vi "copy Data to Array 2D.vi"(4 "error in (no error)":errorcluster, 7 "Data in":refnum<class "Data.lvclass">) -> (0 "error out":errorcluster, 2 "Data Content":sgl[][](array[numeric]), 3 "Data out":refnum<class "Data.lvclass">)   [LabVIEW 2017]
uses:
  C:/Program Files/Thorlabs/SpectralRadar/LabVIEW/2012/user.lib/SpectralRadar.llb/Data.lvclass
  C:/Program Files/Thorlabs/SpectralRadar/LabVIEW/2012/user.lib/SpectralRadar.llb/Data Property Int Selection.ctl
  C:/Program Files/Thorlabs/SpectralRadar/LabVIEW/2012/user.lib/SpectralRadar.llb/get Data Property Int.vi
  SpectralRadar.dll
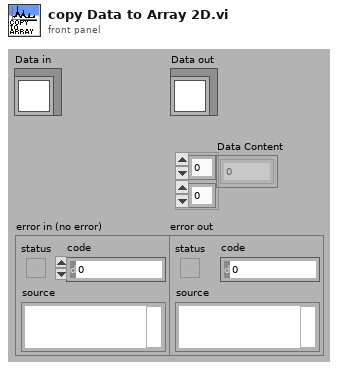
[diagram p1: front panel]
types:
  T1 = typedef "Data.lvclass/Data Property Int Selection.ctl" = enum16{"Dimensions", "Size 1", "Size 2", "Size 3", "Number of Data Points", "Data Size in Bytes", "Bytes per Pixel"}
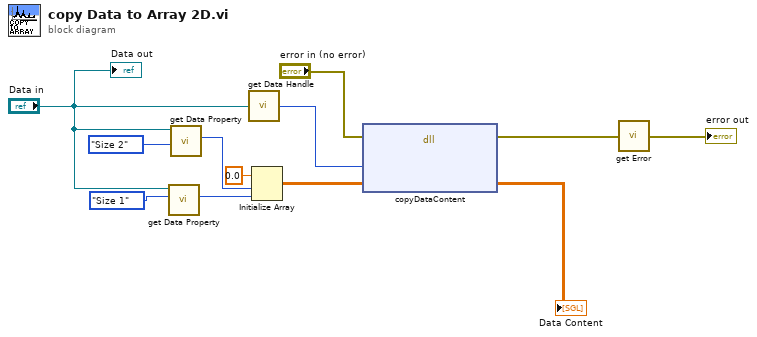
[diagram p0: block diagram]
diagram:
  n1 = call-poly "get Data Property.vi"("Data Property Selection"=Data_Property_Int_Selection."Size 1", "Data"="Data in") -> ("Property Value"=w5:i32)  [unwired: 3 in, 2 out]
  n2 = call-poly "get Data Property.vi"("Data Property Selection"=Data_Property_Int_Selection."Size 2", "Data"="Data in") -> ("Property Value"=w4:i32)  [unwired: 3 in, 2 out]
  n3 = call "get Data Handle.vi"("Data"="Data in") -> ("Handle"=w11:u64)
  n4 = Initialize Array(sgl 0.0 ("element"), w4, w5) -> (w10:sgl[][])
  n5 = dll-call lib="SpectralRadar.dll" fn="copyDataContent"(error in="error in (no error)", "Data Handle"=w11, "Data Content"=w10) -> (error out=w2:errorcluster, "Data Content"=→"Data Content":sgl[][])  [unwired: 4 in, 1 out]
  n6 = call "get Error.vi"("error in (no error)"=w2) -> ("error out"=→"error out":errorcluster)
  "Data out" <- "Data in"
